vi "Set Retardation in nm.vi"(8 "error in (no error)":errorcluster, 10 "Retardance in nm":dbl[unit] min=0.0 max=1.99999e-05 step=1.0000000000000002e-10, 11 "VISA resource name":refnum<visa-resource-name>="COM1") -> (0 "error out":errorcluster, 3 "VISA resource name out":refnum<visa-resource-name>)   [LabVIEW 2017]
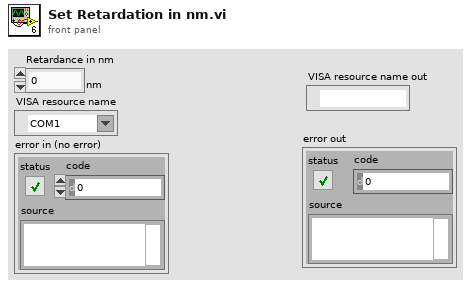
[diagram p1: front panel]
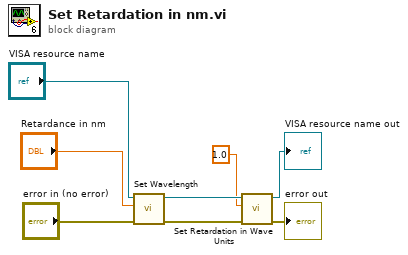
[diagram p0: block diagram]
diagram:
  n1 = call "Set Wavelength.vi"("error in (no error)"="error in (no error)", "wavelength"="Retardance in nm", "VISA resource name"="VISA resource name") -> ("error out"=w7:errorcluster, "VISA resource name out"=w8:refnum<visa-resource-name>)  [unwired: 6 in, 1 out]
  n2 = call "Set Retardation in Wave Units.vi"("VISA resource name"=w8, "fraction of wave"=1.0, "error in (no error)"=w7) -> ("VISA resource name out"=→"VISA resource name out":refnum<visa-resource-name>, "error out"=→"error out":errorcluster)  [unwired: 6 in]
